vi "Get reference.vi"(0 "LV DEV.lvclass":refnum<class "LV DEV.lvclass">, 5 "Vi Path":path, 11 "Error in":errorcluster) -> (4 "LV DEV.lvclass":refnum<class "LV DEV.lvclass">, 15 "Error Out":errorcluster)   [LabVIEW 2016, in "LV DEV.lvclass"]
doc: "Get reference of given VI."
uses:
  Child Classes/LV DEV/LV DEV.lvclass
  D:/MDI Project/source code/Document/Child Classes/LV Doc/LV Doc.lvclass
  LV Doc.lvclass/LV Doc.ctl
  Child Classes/LV DEV/LV DEV.lvclass/LV DEV.ctl
  LV Doc.lvclass
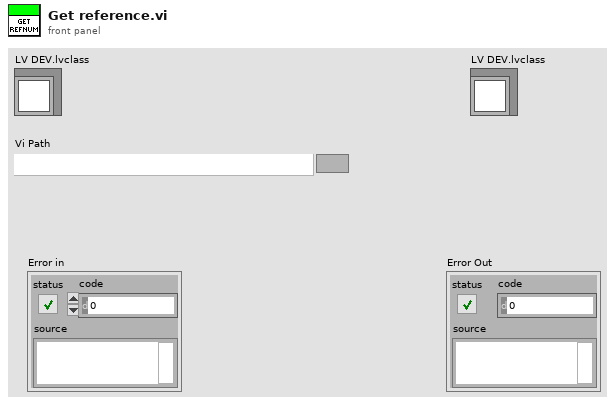
[diagram p1: front panel]
types:
  T1 = enum32{"Invalid", "Standard", "Closed", "Hidden", "Minimized", "Maximized"}
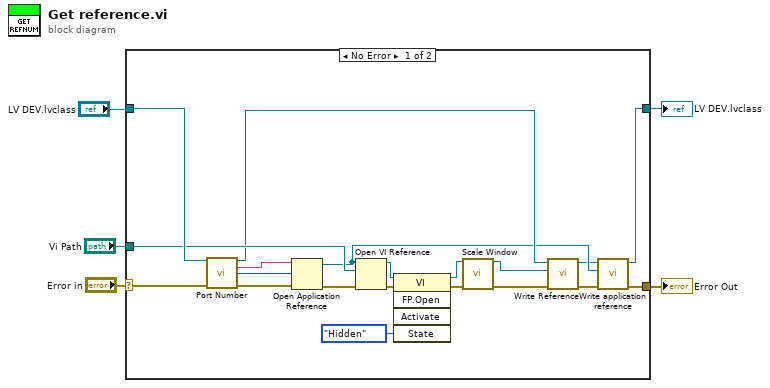
[diagram p0: block diagram]
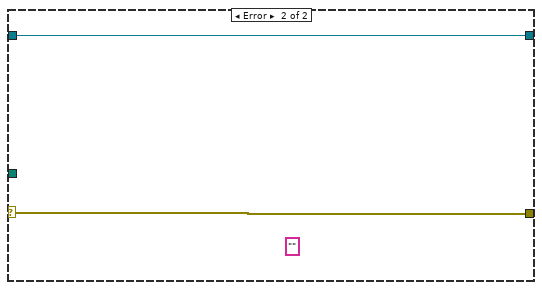
[diagram p2: hidden frame]
diagram:
  n1 = case shown="No Error" "Error in" {
    selector: "Error in" -> [w19 w27]
    tunnel: [w7 w27] -> w4
    tunnel: "Vi Path" -> [w12 _]
    tunnel: "LV DEV.lvclass" -> [w18 w26]
    tunnel: [w8 w26] -> w1
    frame No Error {
      n2 = call "Port Number.vi"("LV DEV.lvclass"=w18, "Error In"=w19) -> ("LV DEV.lvclass"=w11:refnum<class "LV DEV.lvclass">, "Machine name"=w16:string, "Port Number"=w15:u16, "error Out"=w17:errorcluster)  [unwired: 10 in]
      n3 = Open Application Reference(8:w17, 10:w15, 11:w16) -> (0:w23:errorcluster, 3:w10:refnum<vi>)  [unwired: 1 in]
      n4 = Open VI Reference(application reference (local)=w10, vi path=w12, error in (no error)=w23) -> (vi reference=w24:refnum<vi>, error out=w25:errorcluster)  [unwired: 3 in]
      n5 = invoke class="VI" method="FP.Open"(reference=w24, error in=w25, "State"=T1."Hidden") -> (reference out=w20:refnum<vi>, error out=w21:errorcluster)  [unwired: 2 in, 3 out]
      n6 = call "Scale Window.vi"("VI in"=w20, "error in (no error)"=w21) -> ("VI out"=w13:refnum<vi>, "error out"=w14:errorcluster)  [unwired: 12 in]
      n7 = call "Write Reference.vi"("error in (no error)"=w14, "Reference"=w13, "LV Doc in"=w11) -> ("error out"=w6:errorcluster, "LV Doc out"=w9:refnum<class "LV DEV.lvclass">)  [unwired: 7 in]
      n8 = call "Write application reference.vi"("error in (no error)"=w6, "application reference"=w10, "LV DEV in"=w9) -> ("error out"=w7:errorcluster, "LV DEV out"=w8:refnum<class "LV DEV.lvclass">)  [unwired: 7 in]
    }
    frame Error {
      (unwired) "" ("Front Panel.Title")
    }
  }
  "Error Out" <- w4
  "LV DEV.lvclass" <- w1
